vi "Befehle Lesen.vi"(6 "Enum":T1, 8 "error in":errorcluster) -> (0 "error out":errorcluster, 1 "Ausgang für Lesen":string[](array[string]), 2 "Lesebefehl":string[](array[string]), 3 "Schreibbefehl":string[](array[string]))   [LabVIEW 2020, in "Linearisierung v2.lvlib" / "Gasteiler.lvlib" / "HovaCal.lvlib"]
uses:
  HovaCal.lvlib
  Aktion_txt.ctl
  Allgemein/allgemeine Sub-VIs.lvlib
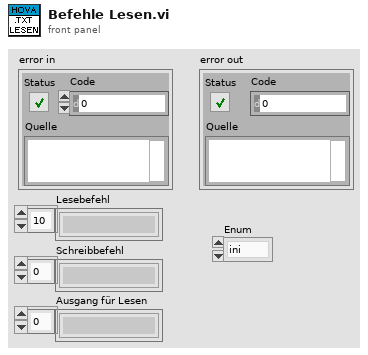
[diagram p1: front panel]
types:
  T1 = typedef "Linearisierung v2.lvlib/Gasteiler.lvlib/HovaCal.lvlib/Aktion_txt.ctl" = enum16{"ini", "lesen"}
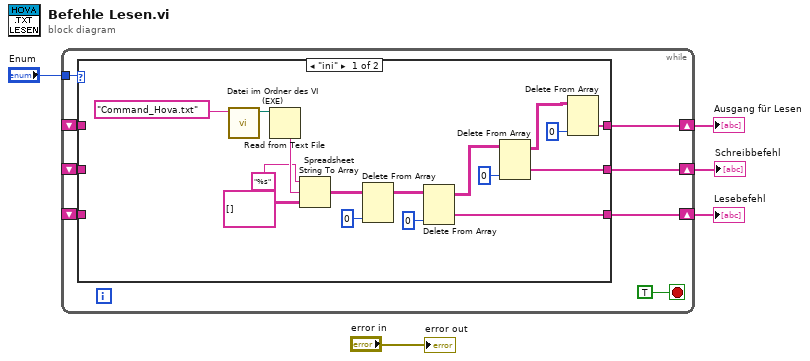
[diagram p0: block diagram]
diagram:
  n1 = while {
    shift-right: [w10] -> w3
    shift-left: _ -> [w9]
    shift-right: [w11] -> w4
    shift-left: _ -> [w8]
    shift-right: [w12] -> w5
    shift-left: _ -> [w7]
    tunnel: "Enum" -> [w6]
    stop <- TRUE stop-if-true
    n2 = case shown="\"ini\"" w6 {
      tunnel: [w26 w30] -> w12
      tunnel: [w23 w31] -> w11
      tunnel: [w20 w32] -> w10
      tunnel: w9 -> [_ w32]
      tunnel: w8 -> [_ w31]
      tunnel: w7 -> [_ w30]
      frame "ini" {
        n3 = call "Datei im Ordner des VI (EXE).vi"("Dateiname"="Command_Hova.txt") -> ("Dateipfad im Ordner des Haupt-VIs"=w14:path)  [unwired: 8 in, 2 out]
        n4 = Read from Text File(file (use dialog)=w14) -> (text=w19:string)  [unwired: 1 in, 5 out]
        n5 = Spreadsheet String To Array(format string="%s" ("Format-String"), spreadsheet string=w19, array type (2D Dbl)=string[][] []) -> (array=w16:string[][])  [unwired: 1 out]
        n6 = Delete From Array(array=w16, index (col)=0 ("Deaktivierter Index (Spalte)")) -> (array with subset deleted=w28:string[][])  [unwired: 2 in, 1 out]
        n7 = Delete From Array(array=w28, index (col)=0 ("Deaktivierter Index (Spalte)")) -> (deleted portion=w26:string[], array with subset deleted=w25:string[][])  [unwired: 2 in]
        n8 = Delete From Array(array=w25, index (col)=0 ("Deaktivierter Index (Spalte)")) -> (deleted portion=w23:string[], array with subset deleted=w22:string[][])  [unwired: 2 in]
        n9 = Delete From Array(array=w22, index (col)=0 ("Deaktivierter Index (Spalte)")) -> (deleted portion=w20:string[])  [unwired: 2 in, 1 out]
      }
      frame "lesen", Default {
      }
    }
  }
  "Lesebefehl" <- w5
  "Schreibbefehl" <- w4
  "Ausgang für Lesen" <- w3
  "error out" <- "error in"
